vi "testing.vi"() -> ()   [LabVIEW 2015]
panel:
  out "x+y":dbl
  in  "Numeric 2":dbl
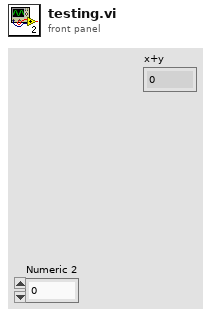
[diagram p1: front panel]
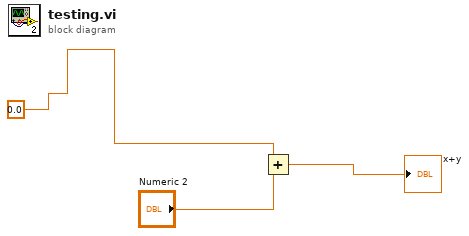
[diagram p0: block diagram]
diagram:
  n1 = Add(x="Numeric 2", y=0.0) -> (x+y=→"x+y":dbl)
